vi "FG-Stop.vi"(8 "error in":errorcluster, 11 "Config. params. ref. in":refnum<data-value>) -> (0 "error IO":errorcluster, 3 "Config. params. ref.":refnum<data-value>)   [LabVIEW 2013, in "CameraVision.lvlib" / "CV-Configuration.lvclass"]
uses:
  CV-Configuration.lvclass
  UI/Module-states.ctl
  CV-Configuration.lvclass/CV-Configuration.ctl
  Read Framegrabber DLL file.vi
  Read BoardHandle.vi
  Read Camport array.vi
  Write Camera status.vi
  Write Grabber status.vi
  UI/CV-UI.lvclass
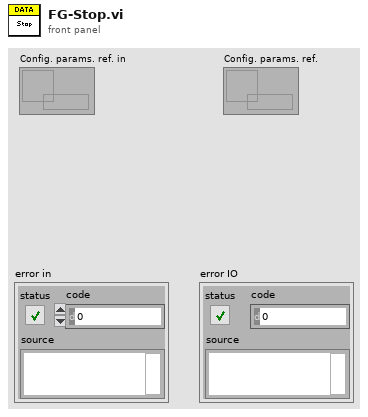
[diagram p1: front panel]
types:
  T1 = typedef "CameraVision.lvlib/CV-UI.lvclass/Module-states.ctl" = enum16{"Inactive", "Active", "Data-loss", "Error", "Simulation", "Synchronizing", "Initialized", "Released"}
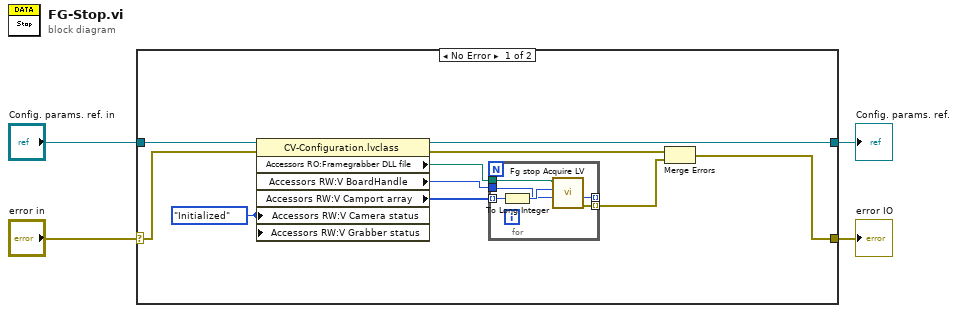
[diagram p0: block diagram]
diagram:
  n1 = case shown="No Error" "error in" {
    selector: "error in" -> [w12 w22]
    tunnel: [w6 w22] -> w4
    tunnel: "Config. params. ref. in" -> [w14 w21]
    tunnel: [w11 w21] -> w1
    frame No Error {
      w5 = Module-states."Initialized" ("Camera status")
      n2 = property class="CV-Configuration.lvclass"(reference=w14, error in=w12, "Accessors RW:V Camera status"=w5, "Accessors RW:V Grabber status"=w5) -> (reference out=w11:refnum<data-value>, error out=w13:errorcluster, "Accessors RO:Framegrabber DLL file"=w10:path, "Accessors RW:V BoardHandle"=w9:u64, "Accessors RW:V Camport array"=w8:u32[])
      n3 = for {
        tunnel: w10 -> [w19]
        tunnel: w9 -> [w17]
        tunnel: w8 -> [w20] mode=indexing
        tunnel: [w15] -> w7 mode=indexing
        tunnel: [w16] -> _ mode=indexing
        n4 = To Long Integer(number=w20) -> (32bit integer=w18:i32)
        n5 = call <userlib>:"Fg stop Acquire LV.vi"("FgAddr"=w17, "CamPort"=w18, "dll path in"=w19) -> ("error out"=w15:errorcluster, "function return"=w16:i32)  [unwired: 2 in, 1 out]
      }
      n6 = Merge Errors(w13, w7) -> (w6:errorcluster)
    }
    frame Error {
    }
  }
  "error IO" <- w4
  "Config. params. ref." <- w1
